vi "Écrire Cooler.vi"(10 "Framework d'acteur:Objet ajoutant des msgs à la file":refnum<class "Message Enqueuer.lvclass">, 11 "Cooler UI with Events en entrée":refnum<class "Cooler UI with Events.lvclass">) -> (3 "Cooler UI with Events en sortie":refnum<class "Cooler UI with Events.lvclass">)   [LabVIEW 2015, in "Cooler UI.lvlib" / "Cooler UI with Events.lvclass"]
uses:
  Cooler UI with Events.lvclass
  <vilib>/ActorFramework/Message Enqueuer/Message Enqueuer.lvclass
  Cooler UI with Events.lvclass/Cooler UI with Events.ctl
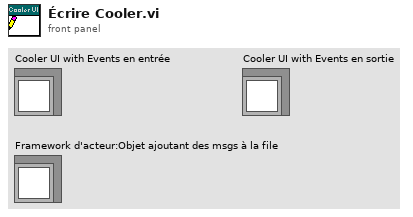
[diagram p1: front panel]
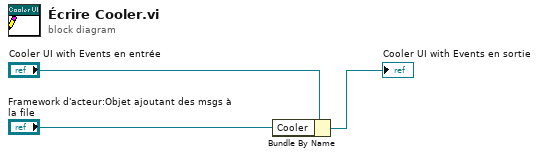
[diagram p0: block diagram]
diagram:
  n1 = Bundle By Name(cluster="Cooler UI with Events en entrée", "Cooler"="Framework d'acteur:Objet ajoutant des msgs à la file") -> (→"Cooler UI with Events en sortie":refnum<class "Cooler UI with Events.lvclass">)
